vi "题目四.vi"() -> ()   [LabVIEW 2017]
uses:
  <vilib>/measure/NI_MABase.lvlib
panel:
  out "大小":i32
  out "最小值":dbl
  out "Y":dbl[](array[numeric])
  out "dt":dbl
  out "signal out":waveform(dbl) caption="信号输出"
  in  "frequency":dbl=10.0 caption="频率" format="%.2p"
  in  "amplitude":dbl=1.0 caption="幅值" format="%.2p"
  in  "phase":dbl caption="相位" format="%.2p"
  in  "sampling info":cluster{"Fs":dbl, "#s":dbl}={"Fs"=1000.0, "#s"=1000.0} caption="采样信息" {"Fs" format="%.2p"}
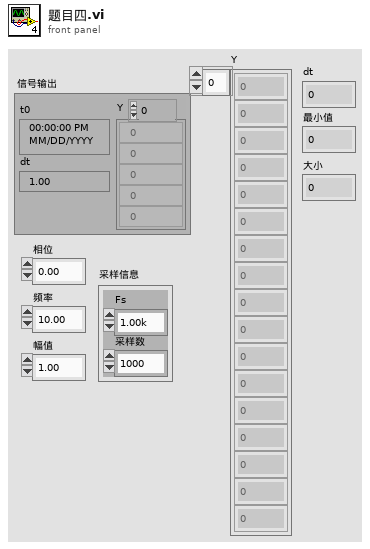
[diagram p1: front panel]
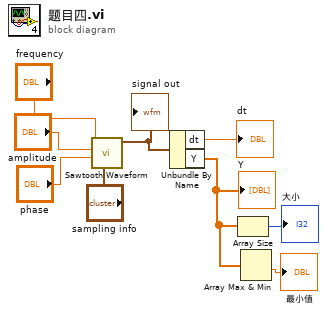
[diagram p0: block diagram]
diagram:
  n1 = call <vilib>:"Sawtooth Waveform.vi"("sampling info"="sampling info", "phase"="phase", "amplitude"="amplitude", "frequency"="frequency") -> ("signal out"=w4:waveform(dbl))  [unwired: 6 in, 1 out]
  "signal out" <- w4
  n2 = Unbundle By Name(w4) -> ("dt"=→"dt":dbl, "Y"=w3:dbl[])
  "Y" <- w3
  n3 = Array Size(array=w3) -> (size(s)=→"大小":i32)
  n4 = Array Max & Min(array=w3) -> (min value=→"最小值":dbl)  [unwired: 3 out]
